vi "Run Test.vi"(8 "error in (no error)":errorcluster, 11 "Test Template in":refnum<class "Short Check.lvclass">) -> (0 "error out":errorcluster, 1 "Positions":i32[](array[numeric]), 2 "Tests Passed":bool[](array[boolean]), 3 "Test Template out":refnum<class "Short Check.lvclass">, 5 "Fail Codes":string[](array[string]))   [LabVIEW 2015, in "Short Check.lvclass"]
uses:
  Short Check.lvclass
  Test Class/Test Class.lvclass
  Classes/Application/Class/Application.lvclass
  Driver Test/Driver Test.lvclass
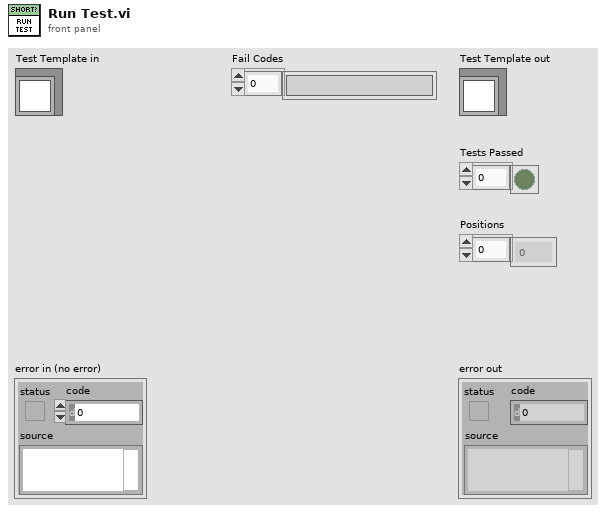
[diagram p1: front panel]
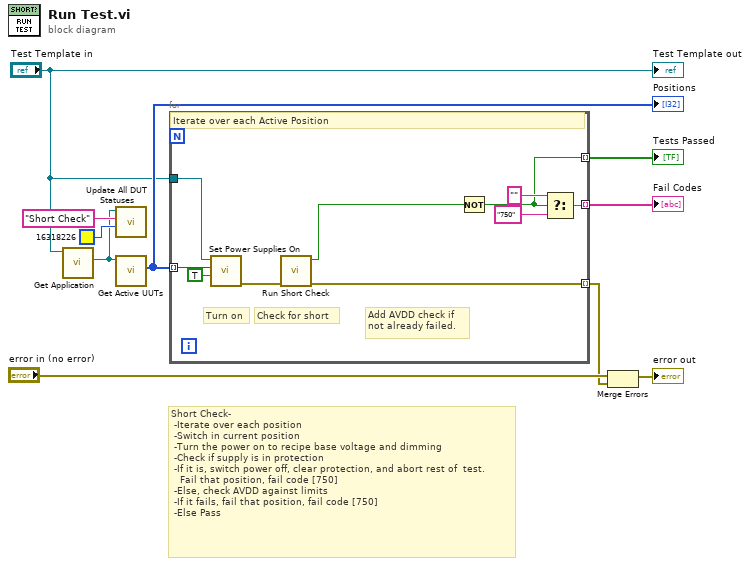
[diagram p0: block diagram]
diagram:
  # "Short Check-\n\t-Iterate over each position\n\t-Switch in current position\n\t-Turn the power on to recipe base voltage and dimming\n\t-Check if supply is in protection\n\t-If it is, switch power off, clear protection, and abort rest of \ttest. \n   Fail that position, fail code [750]\n\t-Else, check AVDD against limits\n\t-If it fails, fail that position, fail code [750]\n\t-Else Pass"
  n1 = call "Get Application.vi"("Test Class in"="Test Template in") -> ("Application.lvlib:Application.lvclass"=w1:refnum<class "Application.lvclass">)  [unwired: 9 in, 1 out]
  n2 = call "Update All DUT Statuses.vi"("BG Color"=u32 16318226, "Message ('')"="Short Check", "Application in"=w1) -> ()  [unwired: 7 in, 2 out]
  n3 = call "Get Active UUTs.vi"("Application in"=w1) -> ("Active Positions"=w4:u32[])  [unwired: 8 in, 2 out]
  "Positions" <- w4
  n4 = for {
    tunnel: w4 -> [w16] mode=indexing
    tunnel: [w20] -> w8 mode=indexing
    tunnel: [w12] -> w7 mode=indexing
    tunnel: [w19] -> w5 mode=indexing
    tunnel: "Test Template in" -> [w17]
    # "Add AVDD check if\nnot already failed."
    # "Turn on"
    # "Check for short"
    # "Iterate over each Active Position"
    n5 = call "Set Power Supplies On.vi"("Power On"=TRUE, "Active Positions"=w16, "Driver Test"=w17) -> ("error out"=w14:errorcluster)  [unwired: 8 in]
    n6 = call "Run Short Check.vi"("error in"=w14) -> ("error out"=w19:errorcluster, "Protected"=w13:bool)  [unwired: 9 in]
    n7 = Not(x=w13) -> (.not. x?=w12:bool)
    n8 = Select(t="", s=w12, f="750") -> (s? t:f=w20:string)
  }
  "Tests Passed" <- w7
  "Fail Codes" <- w8
  n9 = Merge Errors("error in (no error)", w5) -> (→"error out":errorcluster)
  "Test Template out" <- "Test Template in"
